vi "EX 6-2 Thermistor Read.vi"() -> ()   [LabVIEW 2011, in "LabVIEW Interface for Arduino.lvlib"]
doc: "An example that uses an Arduino to read the temperature from a thermistor. The user is able to select the supply voltage, paired resistance, analog input pin and units (C, F, K)."
uses:
  <vilib>/LabVIEW Interface for Arduino/LabVIEW Interface for Arduino.lvlib
panel:
  in  "Paired Resistance (Ohms)":dbl=10000.0
  out "Temperature":dbl(slide) scale=0.0..100.0
  in  "Units":enum16{"Celsius", "Fahrenheit", "Kelvin"}(ring)
  in  "Thermistor AI Pin":u8=1
  in  "Stop":bool
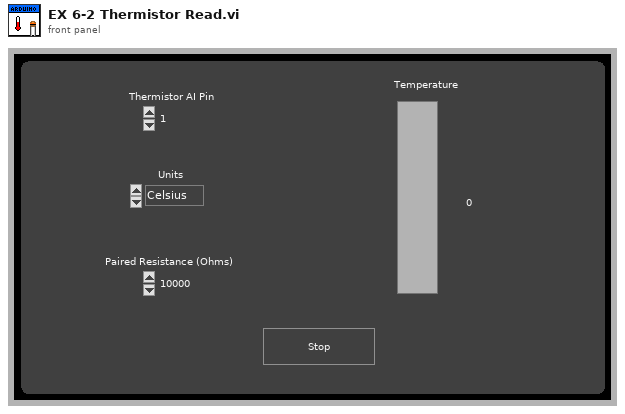
[diagram p1: front panel]
types:
  T1 = typedef "LabVIEW Interface for Arduino.lvlib/Arduino Resource.ctl" = cluster{"VISA resource":refnum<visa-resource-name>, "Board Type":T2, "Connection Type":enum8{"USB / Serial"}, "Bytes Per Packet (15)":u8}
  T2 = typedef "LabVIEW Interface for Arduino.lvlib/Board Type.ctl" = enum16{"Uno", "Dimuelanove w/Atmega 328", "Mega 2560"}
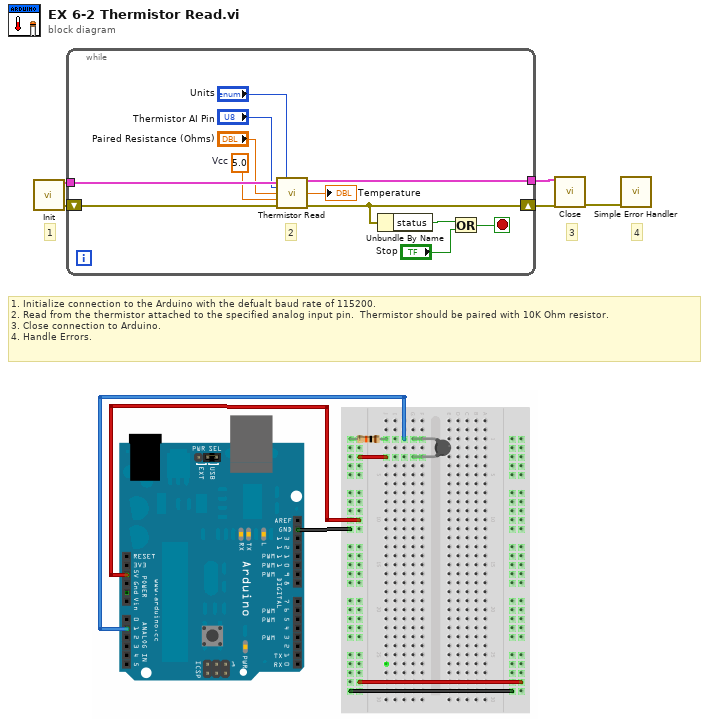
[diagram p0: block diagram]
diagram:
  # "4"
  # "3"
  # "1"
  # "1. Initialize connection to the Arduino with the defualt baud rate of 115200.\n2. Read from the thermistor attached to the specified analog input pin.  Thermistor should be paired with 10K Ohm resistor.\n3. Close connection to Arduino.\n4. Handle Errors."
  n1 = call <vilib>:"Init.vi"() -> ("Arduino Resource"=w5:T1, "error out"=w4:errorcluster)  [unwired: 18 in]
  n2 = while {
    tunnel: w5 -> [w15]
    shift-right: [w10] -> w3
    shift-left: w4 -> [w11]
    tunnel: [w8] -> w1
    stop <- w16 stop-if-true
    w12 = 5.0  # Vcc
    # "2"
    n3 = call <vilib>:"Thermistor Read.vi"("Arduino Resource"=w15, "Units (C)"="Units", "Thermistor AI Pin (0)"="Thermistor AI Pin", "Paired Resistance (10K Ohms)"="Paired Resistance (Ohms)", "Vcc (5 v)"=w12, "error in"=w11) -> ("Arduino Resource"=w8:T1, "Temperature"=→"Temperature":dbl, "error out"=w10:errorcluster)  [unwired: 7 in]
    n4 = Unbundle By Name(w10) -> ("status"=w6:bool)
    n5 = Or(x=w6, y="Stop") -> (x .or. y?=w16:bool)
  }
  n6 = call <vilib>:"Close.vi"("Arduino Resource"=w1, "error in"=w3) -> ("error out"=w2:errorcluster)  [unwired: 13 in]
  n7 = call <vilib>:"Simple Error Handler.vi"("error in (no error)"=w2) -> ()  [unwired: 4 in, 5 out]
